vi "Write Fetch Rooms List and Size Limits Msg.vi"(10 "Guest Manager UI.lvlib:Fetch Rooms List and Size Limits Msg.lvclass":refnum<class "Fetch Rooms List and Size Limits Msg.lvclass">, 11 "Guest Manager UI in":refnum<class "Guest Manager UI.lvclass">) -> (3 "Guest Manager UI out":refnum<class "Guest Manager UI.lvclass">)   [LabVIEW 2023, in "Guest Manager UI.lvlib" / "Guest Manager UI.lvclass"]
uses:
  Guest Manager UI.lvclass
  Guest Manager UI Messages/Fetch Rooms List and Size Limits Msg/Fetch Rooms List and Size Limits Msg.lvclass
  Guest Manager UI.lvclass/Guest Manager UI.ctl
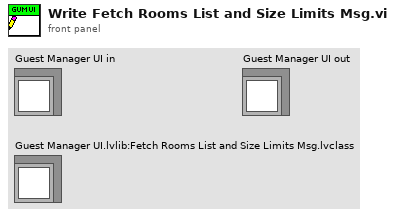
[diagram p1: front panel]
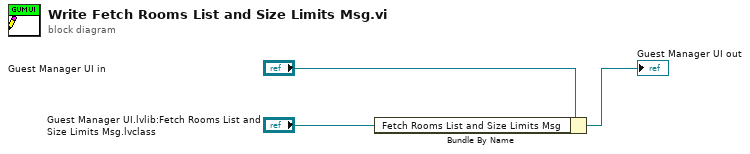
[diagram p0: block diagram]
diagram:
  n1 = Bundle By Name(cluster="Guest Manager UI in", "Fetch Rooms List and Size Limits Msg"="Guest Manager UI.lvlib:Fetch Rooms List and Size Limits Msg.lvclass") -> (→"Guest Manager UI out":refnum<class "Guest Manager UI.lvclass">)
